vi "多参数通讯.vi"(6 "Slave ID":u8=1, 7 "STEP":enum16{"open", "read", "write", "close"}(ring)=enum."read", 8 "Error in":errorcluster caption="Error in (no error)", 9 "values":u16[](array[numeric]), 10 "quantity":u16, 11 "starting address":u16) -> (0 "error out":errorcluster, 2 "输出簇":T1, 3 "Registers":u16[](array[numeric]))   [LabVIEW 2016, in "斯坦道原位多参数.lvlib"]
uses:
  <vilib>/Plasmionique/MB Master/MB_ADU/MB_ADU.lvclass/MB_ADU.ctl
  <vilib>/Plasmionique/MB Master/MB_ADU/Read RX Data.vi
  <vilib>/Plasmionique/MB Master/MB_ADU/Read RX Timestamp.vi
  <vilib>/Plasmionique/MB Master/MB_ADU/Read Slave ID.vi
  <vilib>/Plasmionique/MB Master/MB_ADU/Read TX Data.vi
  <vilib>/Plasmionique/MB Master/MB_ADU/Read TX Timestamp.vi
  <vilib>/Plasmionique/MB Master/MB_Master_Serial/MB_Master_Serial.lvclass
  C:/Program Files (x86)/National Instruments/LabVIEW 2016/vi.lib/Plasmionique/MB Master/MB_Master/MB_Master.lvclass
  <vilib>/Plasmionique/MB Master/MB_ADU/MB_ADU.lvclass
  <vilib>/Plasmionique/MB Master/MB_Master/MB_Master.lvclass
  <vilib>/Plasmionique/MB Master/MB Master.lvlib
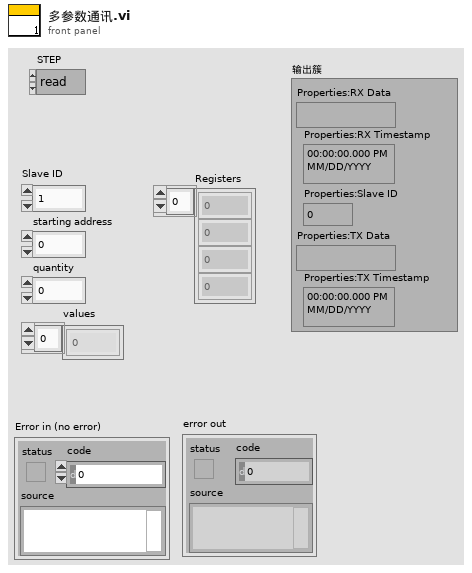
[diagram p1: front panel]
types:
  T1 = cluster{"Properties:RX Data":string, "Properties:RX Timestamp":timestamp, "Properties:Slave ID":u8, "Properties:TX Data":string, "Properties:TX Timestamp":timestamp}
  T2 = cluster{"baud rate (bps)":u32, "stop bits":u16, "parity":u16, "flow control":u16, "timeout":u32, "retries":i32}
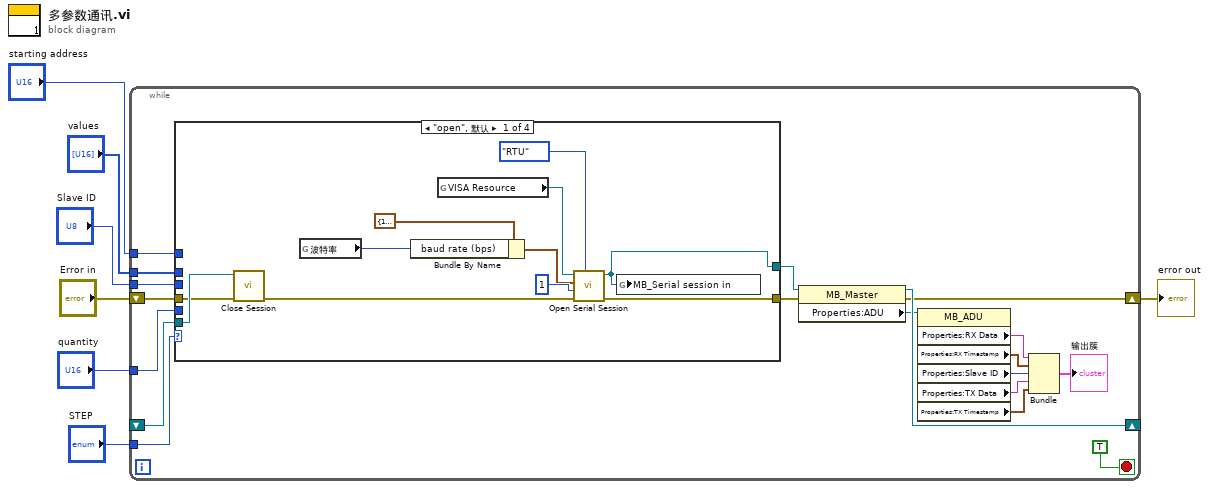
[diagram p0: block diagram]
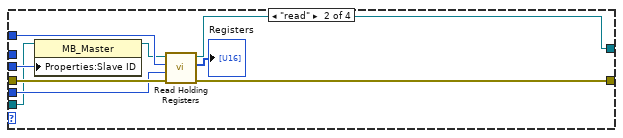
[diagram p2: hidden frame]
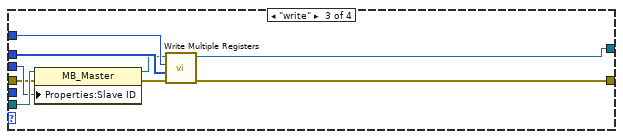
[diagram p3: hidden frame]
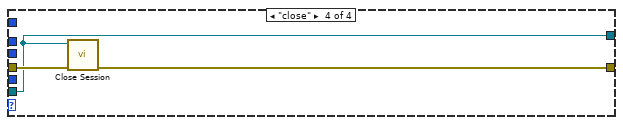
[diagram p4: hidden frame]
diagram:
  n1 = while {
    shift-right: [w20] -> _
    shift-left: _ -> [w26]
    shift-right: [w18] -> w6
    shift-left: "Error in" -> [w25]
    tunnel: "Slave ID" -> [w24]
    tunnel: "starting address" -> [w23]
    tunnel: "quantity" -> [w22]
    tunnel: "STEP" -> [w21]
    tunnel: "values" -> [w11]
    stop <- TRUE stop-if-true
    n2 = case shown="\"open\", 默认" w21 {
      tunnel: w26 -> [w34 w39 w51 w56]
      tunnel: w25 -> [w33 w46 w48 w58]
      tunnel: [w27 w45 w54 w56] -> w8
      tunnel: [w36 w44 w55 w57] -> w19
      tunnel: w24 -> [_ w42 w50 _]
      tunnel: w23 -> [_ w41 w53 _]
      tunnel: w22 -> [_ w40 _ _]
      tunnel: w11 -> [_ _ w52 _]
      frame "open", Default {
        n3 = call-dynamic "Close Session.vi"("error in (no error)"=w33, "MB session in"=w34) -> ("error out"=w32:errorcluster)  [unwired: 9 in]
        n4 = global read "多参数断电保存全局变量.vi" "波特率"() -> (w28:u32)
        n5 = Bundle By Name(cluster=T2 {"baud rate (bps)"=115200, "stop bits"=10, "parity"=0, "flow control"=0, "timeout"=2000, "retries"=1} ("Serial Config"), "baud rate (bps)"=w28) -> (w29:T2)
        n6 = global read "多参数断电保存全局变量.vi" "VISA Resource"() -> (w31:refnum<visa-resource-name>)
        n7 = call <vilib>:"Open Serial Session.vi"("Mode (RTU)"=enum16{"RTU", "ASCII"}."RTU", "Error in"=w32, "Slave ID"=u8 1, "Serial Config"=w29, "VISA Resource"=w31) -> ("Error out"=w36:errorcluster, "MB_Serial session"=w27:refnum<class "MB_Master_Serial.lvclass">)  [unwired: 5 in]
        n8 = global write "多参数全局变量.vi" "MB_Serial session in"(w27) -> ()
      }
      frame "read" {
        n9 = property class="MB_Master"(reference=w39, "Properties:Slave ID"=w42) -> (reference out=w38:refnum<class "MB_Master.lvclass">)  [unwired: 1 in, 1 out]
        n10 = call <vilib>:"Read Holding Registers.vi"("error in (no error)"=w46, "quantity"=w40, "starting address"=w41, "MB session in"=w38) -> ("error out"=w44:errorcluster, "Registers"=→"Registers":u16[], "MB session out"=w45:refnum<class "MB_Master.lvclass">)  [unwired: 5 in]
      }
      frame "write" {
        n11 = property class="MB_Master"(reference=w51, error in=w48, "Properties:Slave ID"=w50) -> (reference out=w49:refnum<class "MB_Master.lvclass">, error out=w47:errorcluster)
        n12 = call <vilib>:"Write Multiple Registers.vi"("error in (no error)"=w47, "values"=w52, "starting address"=w53, "MB session in"=w49) -> ("error out"=w55:errorcluster, "MB session out"=w54:refnum<class "MB_Master.lvclass">)  [unwired: 6 in]
      }
      frame "close" {
        n13 = call-dynamic "Close Session.vi"("error in (no error)"=w58, "MB session in"=w56) -> ("error out"=w57:errorcluster)  [unwired: 9 in]
      }
    }
    n14 = property class="MB_Master"(reference=w8, error in=w19) -> (reference out=w20:refnum<class "MB_Master.lvclass">, error out=w18:errorcluster, "Properties:ADU"=w9:refnum<class "MB_ADU.lvclass">)
    n15 = property class="MB_ADU"(reference=w9) -> ("Properties:RX Data"=w17:string, "Properties:RX Timestamp"=w16:timestamp, "Properties:Slave ID"=w15:u8, "Properties:TX Data"=w14:string, "Properties:TX Timestamp"=w13:timestamp)  [unwired: 1 in, 2 out]
    n16 = Bundle("Properties:RX Data"=w17, "Properties:RX Timestamp"=w16, "Properties:Slave ID"=w15, "Properties:TX Data"=w14, "Properties:TX Timestamp"=w13) -> (→"输出簇":T1)  [unwired: 1 in]
  }
  "error out" <- w6
